vi "Build_URL.vi"(8 "error in":errorcluster, 11 "URL IN":T1) -> (0 "error out":errorcluster, 3 "URL OUT":T1)   [LabVIEW 2016]
uses:
  URL_Data.ctl
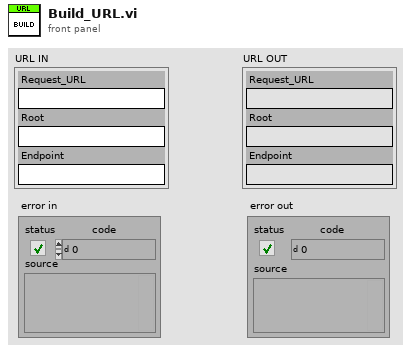
[diagram p1: front panel]
types:
  T1 = typedef "URL_Data.ctl" = cluster{"Root":string, "Endpoint":string, "Request_URL":string}
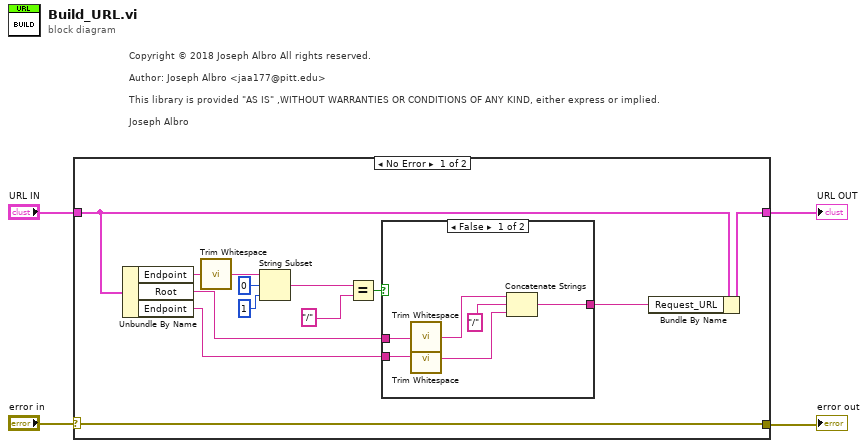
[diagram p0: block diagram]
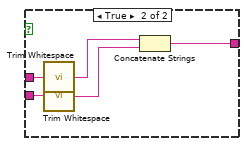
[diagram p2: hidden frame]
diagram:
  # "Copyright © 2018 Joseph Albro All rights reserved.\n\nAuthor: Joseph Albro <jaa177@pitt.edu>\n\nThis library is provided \"AS IS\" ,WITHOUT WARRANTIES OR CONDITIONS OF ANY KIND, either express or implied.\n\nJoseph Albro"
  n1 = case shown="No Error" "error in" {
    selector: "error in" -> [w17 w30]
    tunnel: [w17 w30] -> w3
    tunnel: "URL IN" -> [w7 w29]
    tunnel: [w6 w29] -> w1
    frame No Error {
      n2 = Unbundle By Name(w7) -> ("Endpoint"=w11:string, "Root"=w9:string, "Endpoint"=w8:string)
      n3 = call <vilib>:"Trim Whitespace.vi"("string"=w11) -> ("trimmed string"=w16:string)  [unwired: 1 in]
      n4 = String Subset(string=w16, offset (0)=0, length (rest)=1 ("length (rest)")) -> (substring=w12:string)
      n5 = Equal?(x=w12, y="/") -> (x = y?=w10:bool)
      n6 = case shown="False" w10 {
        tunnel: w9 -> [w23 w27]
        tunnel: w8 -> [w22 w28]
        tunnel: [w18 w24] -> w5
        frame False {
          n7 = call <vilib>:"Trim Whitespace.vi"("string"=w23) -> ("trimmed string"=w20:string)  [unwired: 1 in]
          n8 = call <vilib>:"Trim Whitespace.vi"("string"=w22) -> ("trimmed string"=w19:string)  [unwired: 1 in]
          n9 = Concatenate Strings(w20, "/" ("string"), w19) -> (w18:string)
        }
        frame True {
          n10 = call <vilib>:"Trim Whitespace.vi"("string"=w27) -> ("trimmed string"=w26:string)  [unwired: 1 in]
          n11 = call <vilib>:"Trim Whitespace.vi"("string"=w28) -> ("trimmed string"=w25:string)  [unwired: 1 in]
          n12 = Concatenate Strings(w26, w25) -> (w24:string)
        }
      }
      n13 = Bundle By Name(cluster=w7, "Request_URL"=w5) -> (w6:T1)
    }
    frame Error {
    }
  }
  "error out" <- w3
  "URL OUT" <- w1
